vi "DELETE Template.vi"(8 "error in":errorcluster, 11 "Nominal Client in":refnum<class "Nominal Client.lvclass">) -> (0 "error out":errorcluster, 2 "Response":string, 3 "Nominal Client out":refnum<class "Nominal Client.lvclass">)   [LabVIEW 2020]
doc: "This template lets end users extend the Nominal LabVIEW Client without waiting for Nominal to implement new functionality.\n\nDropping this template onto your block diagram drops the code directly, not a subVI.\n\nSave VIs created from this template in your project source code, not the toolkit source code, as they will be removed when the toolkit updates.\n\nIf you would like to contribute to the Nominal LabVIEW Client toolkit, speak to a member of our team."
uses:
  Nominal Client/Nominal Client.lvclass
  Nominal Client/Nominal Client.lvclass/Nominal Client.ctl
  Nominal Client/create.authorization_header.vi
  Nominal Client/trace.payload_sent.vi
  Nominal Client/trace.payload_received.vi
  Nominal Client/error.vi
  Nominal Client/api_token.get.vi
  Nominal Client/trace.calling_method.vi
  <vilib>/JDP Science/JDP Science Common Utilities/Trim Whitespace__JDP.vi
  <vilib>/AdvancedString/1D String Array to Delimited String.vi
  Nominal Client/error.vi/859f8e04-e495-489b-b5b4-7ac163f56130.vi
  <vilib>/Utility/libraryn.llb/Get File Extension.vi
  Nominal Client/log_file.write.vi
  submodules/reqwest-labview/lv-src/reqwest/get.vi
  <vilib>/JDP Science/JSONtext/Get all Object Items.vi
  <vilib>/Utility/error.llb/Error Cluster From Error Code.vi
  <vilib>/JDP Science/JSONtext/JSON text to Variant.vi
  <vilib>/JDP Science/JSONtext/LVClass Serializer/JSONtext LVClass Serializer.lvclass
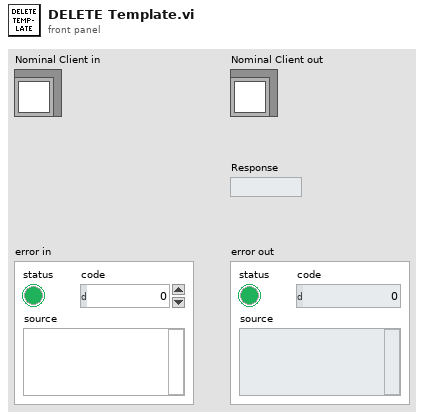
[diagram p1: front panel]
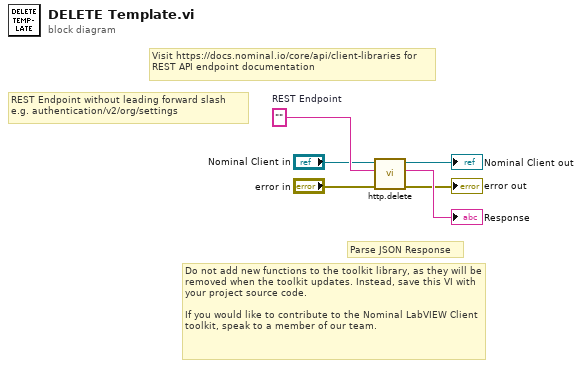
[diagram p0: block diagram]
diagram:
  w6 = ""  # REST Endpoint
  # "Do not add new functions to the toolkit library, as they will be removed when the toolkit updates. Instead, save this VI with your project source code.\n\nIf you would like to contribute to the Nominal LabVIEW Client toolkit, speak to a member of our team."
  # "Parse JSON Response"
  # "REST Endpoint without leading forward slash\ne.g. authentication/v2/org/settings"
  # "Visit https://docs.nominal.io/core/api/client-libraries for REST API endpoint documentation"
  n1 = call "http.delete.vi"("error in"="error in", "Path"=w6, "Nominal Client in"="Nominal Client in") -> ("error out"=→"error out":errorcluster, "Response"=→"Response":string, "Nominal Client out"=→"Nominal Client out":refnum<class "Nominal Client.lvclass">)  [unwired: 6 in]
